vi "sub_DTMF_To_Bitstream.vi"(9 "Packet\nMessage Length (bits)":i32, 11 "DTMF Settings":T1={"Phone Number"="", "Dial Tone"=FALSE, "Quantization Level"=4, "\nGray Encoding"=FALSE} {"Quantization Level" items=["2"=2, "4"=4, "8"=8, "16"=16]}) -> (0 "TX DTMF Signal":dbl[][](array[numeric]), 1 "File Length (bits)":i32, 3 "message bitstream":i8[](array[numeric]), 4 "Number of Packets":i32)   [LabVIEW 2011]
panel:
  out "Array":i8[][](array[numeric])
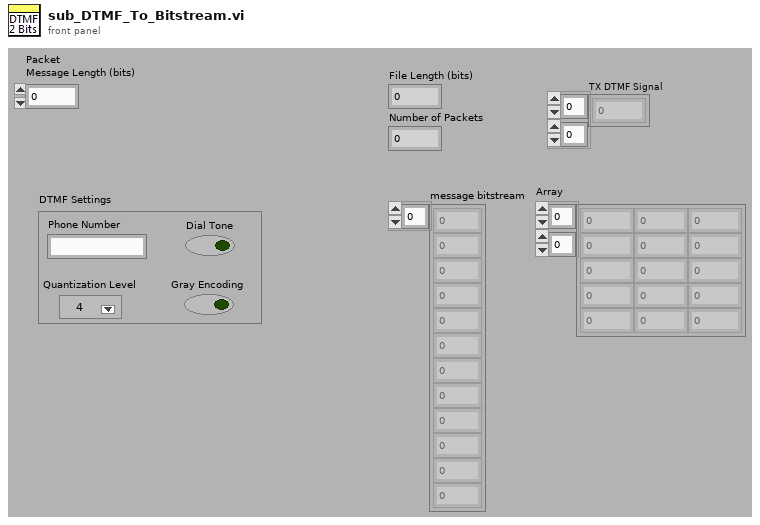
[diagram p1: front panel]
types:
  T1 = cluster{"Phone Number":string, "Dial Tone":bool, "Quantization Level":u16, "\nGray Encoding":bool}
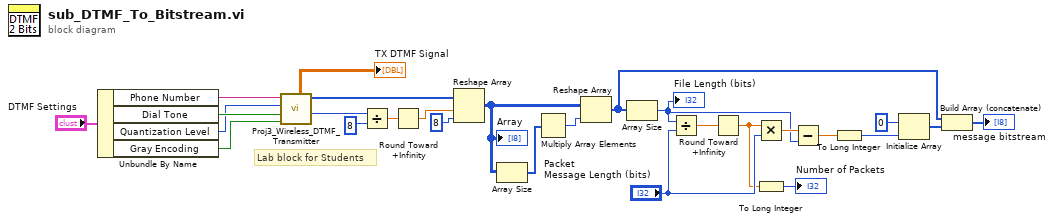
[diagram p0: block diagram]
diagram:
  # "Lab block for Students"
  n1 = Unbundle By Name("DTMF Settings") -> ("Phone Number"=w5:string, "Dial Tone"=w4:bool, "Quantization Level"=w3:u16, "Gray Encoding"=w2:bool)
  n2 = call "Proj3_Wireless_DTMF_Transmitter.vi"("Gray Bit Encoding"=w2, "Dial Tone"=w4, "Quantization Level"=w3, "Phone # String"=w5) -> ("bitLength"=w7:i32, "TXbitStream"=w8:i8[], "TX DTMF Signal"=→"TX DTMF Signal":dbl[][])  [unwired: 1 in, 2 out]
  n3 = Divide(x=w7, y=8) -> (x/y=w12:dbl)
  n4 = Round Toward +Infinity(x=w12) -> (ceil(x): smallest int >= x=w11:dbl)
  n5 = Reshape Array(w8, w11, 8 ("dimension size")) -> (w9:i8[][])
  "Array" <- w9
  n6 = Array Size(array=w9) -> (size(s)=w27:i32[])
  n7 = Multiply Array Elements(1:w27) -> (0:w26:i32)
  n8 = Reshape Array(w9, w26) -> (w16:i8[])
  n9 = Array Size(array=w16) -> (size(s)=w22:i32)
  "File Length (bits)" <- w22
  n10 = Divide(x=w22, y="Packet\nMessage Length (bits)") -> (x/y=w24:dbl)
  n11 = Round Toward +Infinity(x=w24) -> (ceil(x): smallest int >= x=w19:dbl)
  n12 = Multiply(x=w19, y="Packet\nMessage Length (bits)") -> (x*y=w23:dbl)
  n13 = To Long Integer(number=w19) -> (32bit integer=→"Number of Packets":i32)
  n14 = Subtract(x=w23, y=w22) -> (x-y=w21:dbl)
  n15 = To Long Integer(number=w21) -> (32bit integer=w17:i32)
  n16 = Initialize Array(i8 0 ("element"), w17) -> (w15:i8[])
  n17 = Build Array (concatenate)(w16, w15) -> (→"message bitstream":i8[])
